vi "XML.SaveAsPrettyPrint.vi"(8 "error in (no error)":errorcluster, 11 "XML file path":path) -> (0 "error out":errorcluster)   [LabVIEW 2019, in "Tools.lvlib"]
doc: "This VI saves <b>XML file</b> with a Pretty Print option. It does not change any data inside. It needs to be used because LibXML does not save xml files with Pretty Print option, so this one uses NI XML library."
uses:
  <vilib>/xml/Load XML File.vi
  <vilib>/xml/Close Reference(Node).vi
  Tools.lvlib
  <resource>/objmgr/DOMUserDefRef.rc
  <vilib>/xml/NI_XML.lvlib
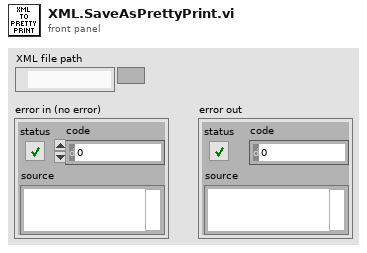
[diagram p1: front panel]
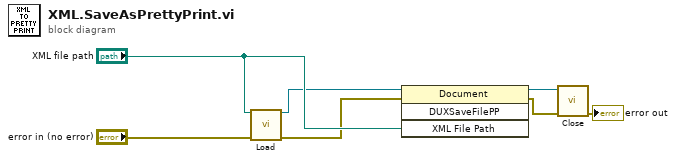
[diagram p0: block diagram]
diagram:
  n1 = call-poly <vilib>:"Load.vi"("path to XML document"="XML file path", "error in (no error)"="error in (no error)") -> ("DOM document out"=w6:refnum<k20>, "error out"=w5:errorcluster)  [unwired: 11 in, 1 out]
  n2 = invoke class="Document" method="DUXSaveFilePP"(reference=w6, error in=w5, "XML File Path"="XML file path") -> (reference out=w1:refnum<k20>, error out=w2:errorcluster)  [unwired: 1 in, 2 out]
  n3 = call-poly <vilib>:"Close.vi"("error in (no error)"=w2, "node"=w1) -> ("error out"=→"error out":errorcluster)  [unwired: 7 in]
